vi "RTP_RTSP - READ PAYLOAD - METHOD.vi"(0 "RTSP Session":T2, 7 "H264 NAL unit":T1, 9 "timeout ms (1000)":i32=1000, 11 "error in (no error)":errorcluster) -> (4 "RTSP Session 2":T2, 6 "timestamp":u32, 8 "H264 NAL unit 2":T1, 15 "error out":errorcluster)   [LabVIEW 2014]
uses:
  RTSP Session.ctl
  H264 NAL unit.ctl
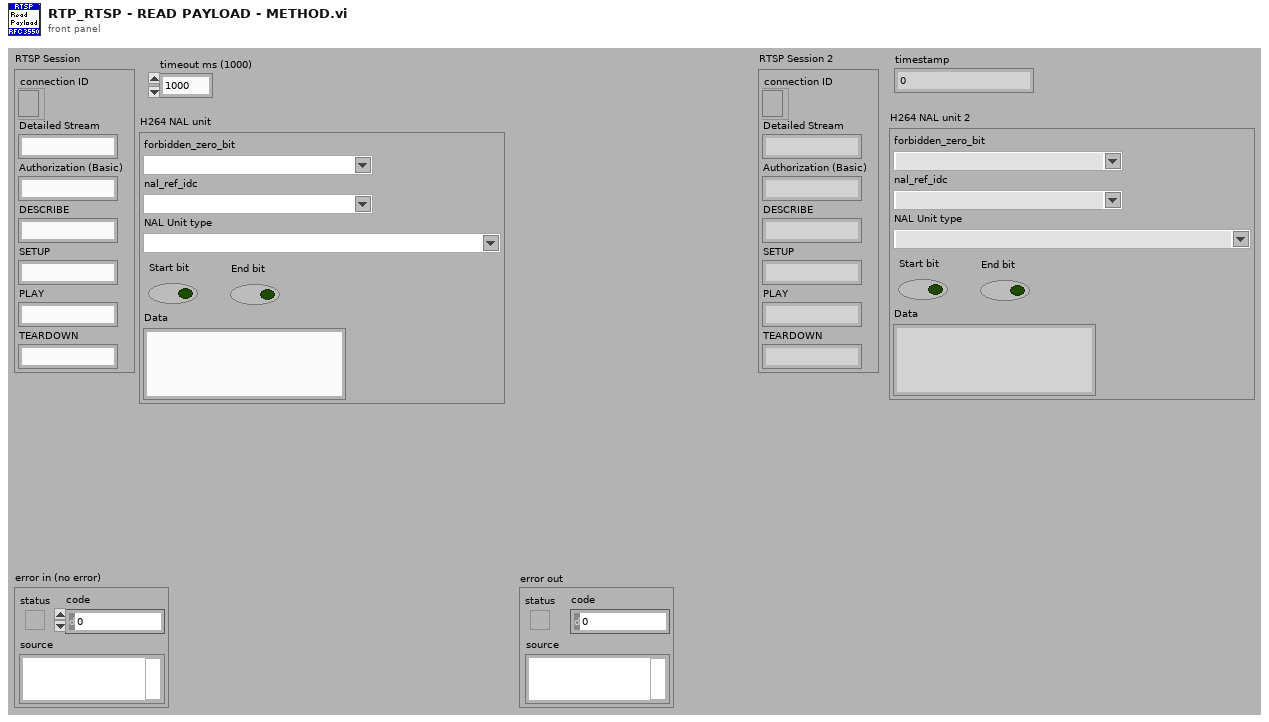
[diagram p1: front panel]
types:
  T1 = typedef "H264 NAL unit.ctl" = cluster{"forbidden_zero_bit":string, "nal_ref_idc":string, "NAL Unit type":string, "Start bit":bool, "End bit":bool, "Data":string}
  T2 = typedef "RTSP Session.ctl" = cluster{"connection ID":refnum<k5>, "Authorization (Basic)":string, "Detailed Stream":string, "DESCRIBE":string, "SETUP":string, "PLAY":string, "TEARDOWN":string}
  T3 = cluster{"Version":string, "Padding":string, "extension (X)":string, "CSRC count (CC)":string, "marker (M)":string, "Payload type":string, "Sequence number":u32, "timestamp":u32, "SSRC":u32}
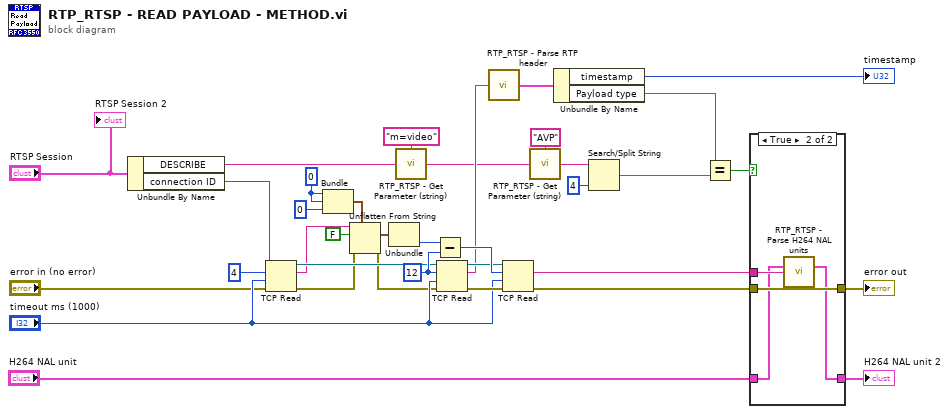
[diagram p0: block diagram]
diagram:
  w28 = 12 ("bytes to read")
  w21 = u8 0
  n1 = Unbundle By Name("RTSP Session") -> ("DESCRIBE"=w14:string, "connection ID"=w26:refnum<k5>)
  n2 = TCP Read(connection ID=w26, bytes to read=4, error in (no error)="error in (no error)", 9:"timeout ms (1000)") -> (connection ID out=w27:refnum<k5>, data out=w22:string, error out=w19:errorcluster)  [unwired: 1 in]
  n3 = Bundle(w21, w21, u16 0) -> (w32:cluster{u8, u8, u16})  [unwired: 1 in]
  n4 = Unflatten From String(type=w32, binary string=w22, data includes array or string size? (T)=FALSE, error in (no error)=w19) -> (value=w34:cluster{u8, u8, u16}, error out=w18:errorcluster)  [unwired: 1 in, 1 out]
  n5 = Unbundle(w34) -> (w20:u16)  [unwired: 2 out]
  n6 = call "RTP_RTSP - Get Parameter (string).vi"("Name"="m=video", "Data"=w14) -> ("Parameter"=w12:string)  [unwired: 13 in]
  n7 = Subtract(x=w20, y=w28) -> (x-y=w31:i32)
  n8 = TCP Read(connection ID=w27, bytes to read=w28, error in (no error)=w18, 9:"timeout ms (1000)") -> (connection ID out=w29:refnum<k5>, data out=w17:string, error out=w30:errorcluster)  [unwired: 1 in]
  n9 = call "RTP_RTSP - Parse RTP header.vi"("RTP Packet"=w17) -> ("RTP Header"=w16:T3)  [unwired: 14 in]
  n10 = TCP Read(connection ID=w29, bytes to read=w31, error in (no error)=w30, 9:"timeout ms (1000)") -> (data out=w15:string, error out=w4:errorcluster)  [unwired: 1 in, 1 out]
  n11 = call "RTP_RTSP - Get Parameter (string).vi"("Name"="AVP", "Data"=w12) -> ("Parameter"=w10:string)  [unwired: 13 in]
  n12 = Unbundle By Name(w16) -> ("timestamp"=→"timestamp":u32, "Payload type"=w8:string)
  n13 = Search/Split String(string=w10, offset (0)=4) -> (match + rest of string=w7:string)  [unwired: 1 in, 2 out]
  n14 = Equal?(x=w8, y=w7) -> (x = y?=w6:bool)
  n15 = case shown="True" w6 {
    tunnel: w15 -> [_ w42]
    tunnel: [w38 w41] -> w5
    tunnel: w4 -> [w38 w41]
    tunnel: "H264 NAL unit" -> [w37 w40]
    tunnel: [w37 w39] -> w2
    frame False {
    }
    frame True {
      n16 = call "RTP_RTSP - Parse H264 NAL units.vi"("H264 NAL unit"=w40, "New Payload"=w42) -> ("H264 NAL unit 2"=w39:T1)  [unwired: 13 in]
    }
  }
  "error out" <- w5
  "H264 NAL unit 2" <- w2
  "RTSP Session 2" <- "RTSP Session"
